vi "Test GPU FFT.vi"() -> ()   [LabVIEW 2018]
panel:
  out "Waveform Chart":dbl(graph)
  out "time":dbl
  out "i":i32
  out "h_trimmed_signal":sgl[](graph)
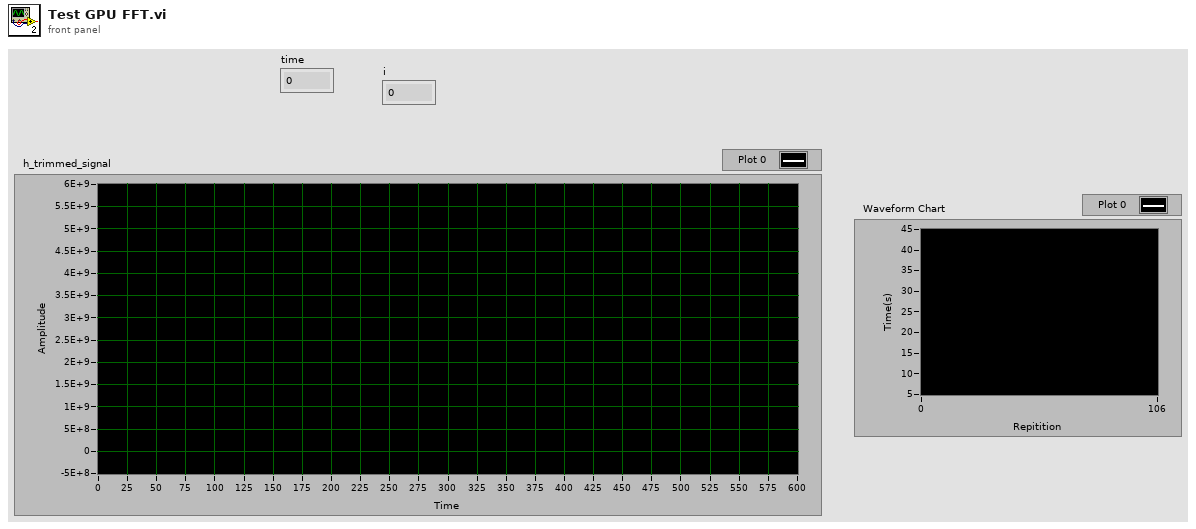
[diagram p1: front panel]
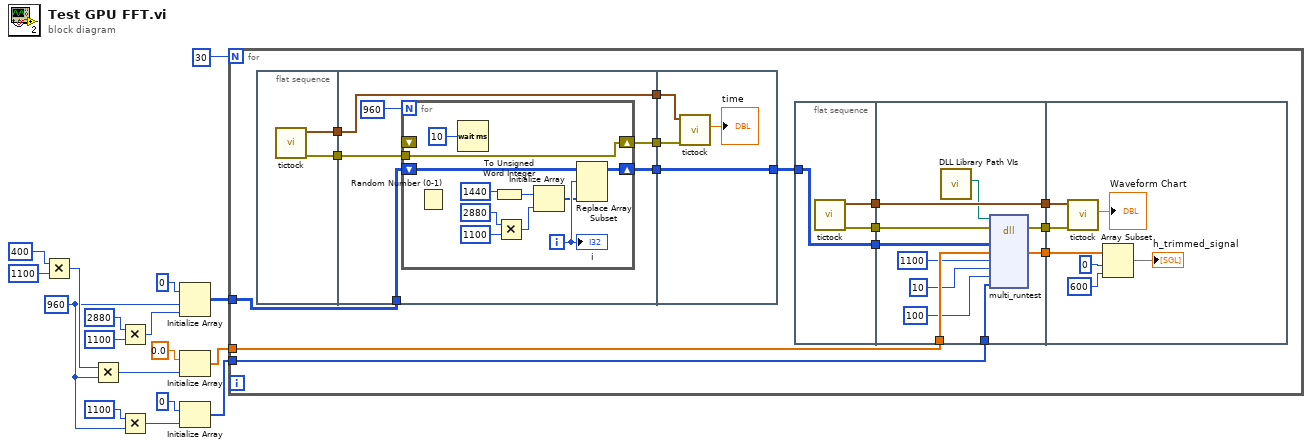
[diagram p0: block diagram]
diagram:
  w2 = 960 ("dimension size")
  n1 = Multiply(x=400, y=1100) -> (x*y=w12:i32)
  n2 = Multiply(x=w12, y=w2) -> (x*y=w11:i32)
  n3 = Multiply(x=u32 2880 ("element"), y=u32 1100 ("element")) -> (x*y=w14:u32)
  n4 = Multiply(x=1100, y=w2) -> (x*y=w4:i32)
  n5 = Initialize Array(u16 0 ("element"), w2, w14) -> (w1:u16[][])
  n6 = Initialize Array(sgl 0.0 ("element"), w11) -> (w7:sgl[])
  n7 = Initialize Array(0 ("element"), w4) -> (w3:i32[])
  n8 = for {
    N: 30 -> [_]
    tunnel: w7 -> [w26]
    tunnel: w3 -> [w25]
    tunnel: w1 -> [w19]
    n9 = flat-sequence {
      tunnel: [w34] -> w24
      tunnel: [w33] -> w23
      tunnel: [w40] -> w22
      tunnel: w24 -> [w40]
      tunnel: w23 -> [w39]
      tunnel: [w38] -> w21
      tunnel: w19 -> [w37]
      tunnel: [w36] -> w20
      tunnel: w22 -> [w55]
      tunnel: w21 -> [w54]
      tunnel: w20 -> [w52]
      tunnel: [w52] -> w18
      frame #0 {
        n10 = call "tictock.vi"() -> ("error out"=w33:errorcluster, "seconds since 1Jan1904"=w34:timestamp)  [unwired: 9 in, 1 out]
      }
      frame #1 {
        n11 = for {
          N: 960 ("x") -> [_]
          tunnel: w39 -> [w51]
          shift-right: [w51] -> w38
          shift-left: _ -> [_]
          shift-right: [w49] -> w36
          shift-left: w37 -> [w50]
          i -> [w48]
          n12 = Random Number (0-1)() -> ()  [unwired: 1 out]
          n13 = Wait (ms)(milliseconds to wait=u32 10) -> ()  [unwired: 1 out]
          n14 = To Unsigned Word Integer(number=u32 1440 ("element")) -> (unsigned 16bit integer=w42:u16)
          n15 = Multiply(x=u32 2880 ("element"), y=u32 1100 ("element")) -> (x*y=w46:u32)
          n16 = Initialize Array(w42, w46) -> (w43:u16[])
          n17 = Replace Array Subset(array=w50, new element=w43, index (row)=w48) -> (w49:u16[][])  [unwired: 1 in]
          "i" <- w48
        }
      }
      frame #2 {
        n18 = call "tictock.vi"("error in (no error)"=w54, "seconds since 1Jan1904 2"=w55) -> ("Numeric"=→"time":dbl)  [unwired: 7 in, 2 out]
      }
    }
    n19 = flat-sequence {
      tunnel: [w58] -> w32
      tunnel: [w57] -> w31
      tunnel: [w56] -> w30
      tunnel: w18 -> [w56]
      tunnel: w32 -> [w69]
      tunnel: w31 -> [w67]
      tunnel: w30 -> [w66]
      tunnel: w26 -> [w65]
      tunnel: [w64] -> w29
      tunnel: [w68] -> w28
      tunnel: [w69] -> w27
      tunnel: w25 -> [w60]
      tunnel: w29 -> [w72]
      tunnel: w28 -> [w74]
      tunnel: w27 -> [w73]
      frame #0 {
        n20 = call "tictock.vi"() -> ("error out"=w57:errorcluster, "seconds since 1Jan1904"=w58:timestamp)  [unwired: 9 in, 1 out]
      }
      frame #1 {
        n21 = call "DLL Library Path VIs.vi"() -> ("GPUFFT"=w59:path)  [unwired: 9 in, 2 out]
        n22 = dll-call lib="C:/Project/SerialSectOCT - FFT GPU/SerialSectOCT/Labview Software/DLL/CUDA_FFT_100-1.dll" fn="multi_runtest"(path in=w59, error in=w67, "h_signal"=w66, "h_trimmed_signal"=w65, "num_aline"=1100, "start"=10, "depth"=100, "curve"=w60) -> (error out=w68:errorcluster, "h_trimmed_signal"=w64:sgl[])  [unwired: 7 in, 1 out]
      }
      frame #2 {
        n23 = call "tictock.vi"("error in (no error)"=w74, "seconds since 1Jan1904 2"=w73) -> ("Numeric"=→"Waveform Chart":dbl)  [unwired: 7 in, 2 out]
        n24 = Array Subset(array=w72, index=0, length=600) -> (→"h_trimmed_signal":sgl[])
      }
    }
  }
